vi "多通道CAN FD回读.vi"(8 "错误输入（无错误）":errorcluster, 10 "Delay Time (s)":dbl=0.2 format="%#_13g", 11 "CAN通道in":u16[](array[numeric])=[81, 82, 83]) -> (0 "错误输出":errorcluster, 3 "报文数组":string[](array[string]))   [LabVIEW 2021]
panel:
  out "function return":u32
  in  "MessageBuffer in":T1 {"DATA"."[0]" format="%x"; "DATA"."[1]" format="%x"; "DATA"."[2]" format="%x"; "DATA"."[3]" format="%x"; "DATA"."[4]" format="%x"; "DATA"."[5]" format="%x"; "DATA"."[6]" format="%x"; "DATA"."[7]" format="%x"; "DATA"."[8]" format="%x"; "DATA"."[9]" format="%x"; "DATA"."[10]" format="%x"; "DATA"."[11]" format="%x"; "DATA"."[12]" format="%x"; "DATA"."[13]" format="%x"; "DATA"."[14]" format="%x"; "DATA"."[15]" format="%x"; "DATA"."[16]" format="%x"; "DATA"."[17]" format="%x"; "DATA"."[18]" format="%x"; "DATA"."[19]" format="%x"; "DATA"."[20]" format="%x"; "DATA"."[21]" format="%x"; "DATA"."[22]" format="%x"; "DATA"."[23]" format="%x"; "DATA"."[24]" format="%x"; "DATA"."[25]" format="%x"; "DATA"."[26]" format="%x"; "DATA"."[27]" format="%x"; "DATA"."[28]" format="%x"; "DATA"."[29]" format="%x"; "DATA"."[30]" format="%x"; "DATA"."[31]" format="%x"; "DATA"."[32]" format="%x"; "DATA"."[33]" format="%x"; "DATA"."[34]" format="%x"; "DATA"."[35]" format="%x"; "DATA"."[36]" format="%x"; "DATA"."[37]" format="%x"; "DATA"."[38]" format="%x"; "DATA"."[39]" format="%x"; "DATA"."[40]" format="%x"; "DATA"."[41]" format="%x"; "DATA"."[42]" format="%x"; "DATA"."[43]" format="%x"; "DATA"."[44]" format="%x"; "DATA"."[45]" format="%x"; "DATA"."[46]" format="%x"; "DATA"."[47]" format="%x"; "DATA"."[48]" format="%x"; "DATA"."[49]" format="%x"; "DATA"."[50]" format="%x"; "DATA"."[51]" format="%x"; "DATA"."[52]" format="%x"; "DATA"."[53]" format="%x"; "DATA"."[54]" format="%x"; "DATA"."[55]" format="%x"; "DATA"."[56]" format="%x"; "DATA"."[57]" format="%x"; "DATA"."[58]" format="%x"; "DATA"."[59]" format="%x"; "DATA"."[60]" format="%x"; "DATA"."[61]" format="%x"; "DATA"."[62]" format="%x"; "DATA"."[63]" format="%x"; "ID" format="%.0x"; "MSGTYPE" format="%.0x"; "DLC" format="%.0x"}
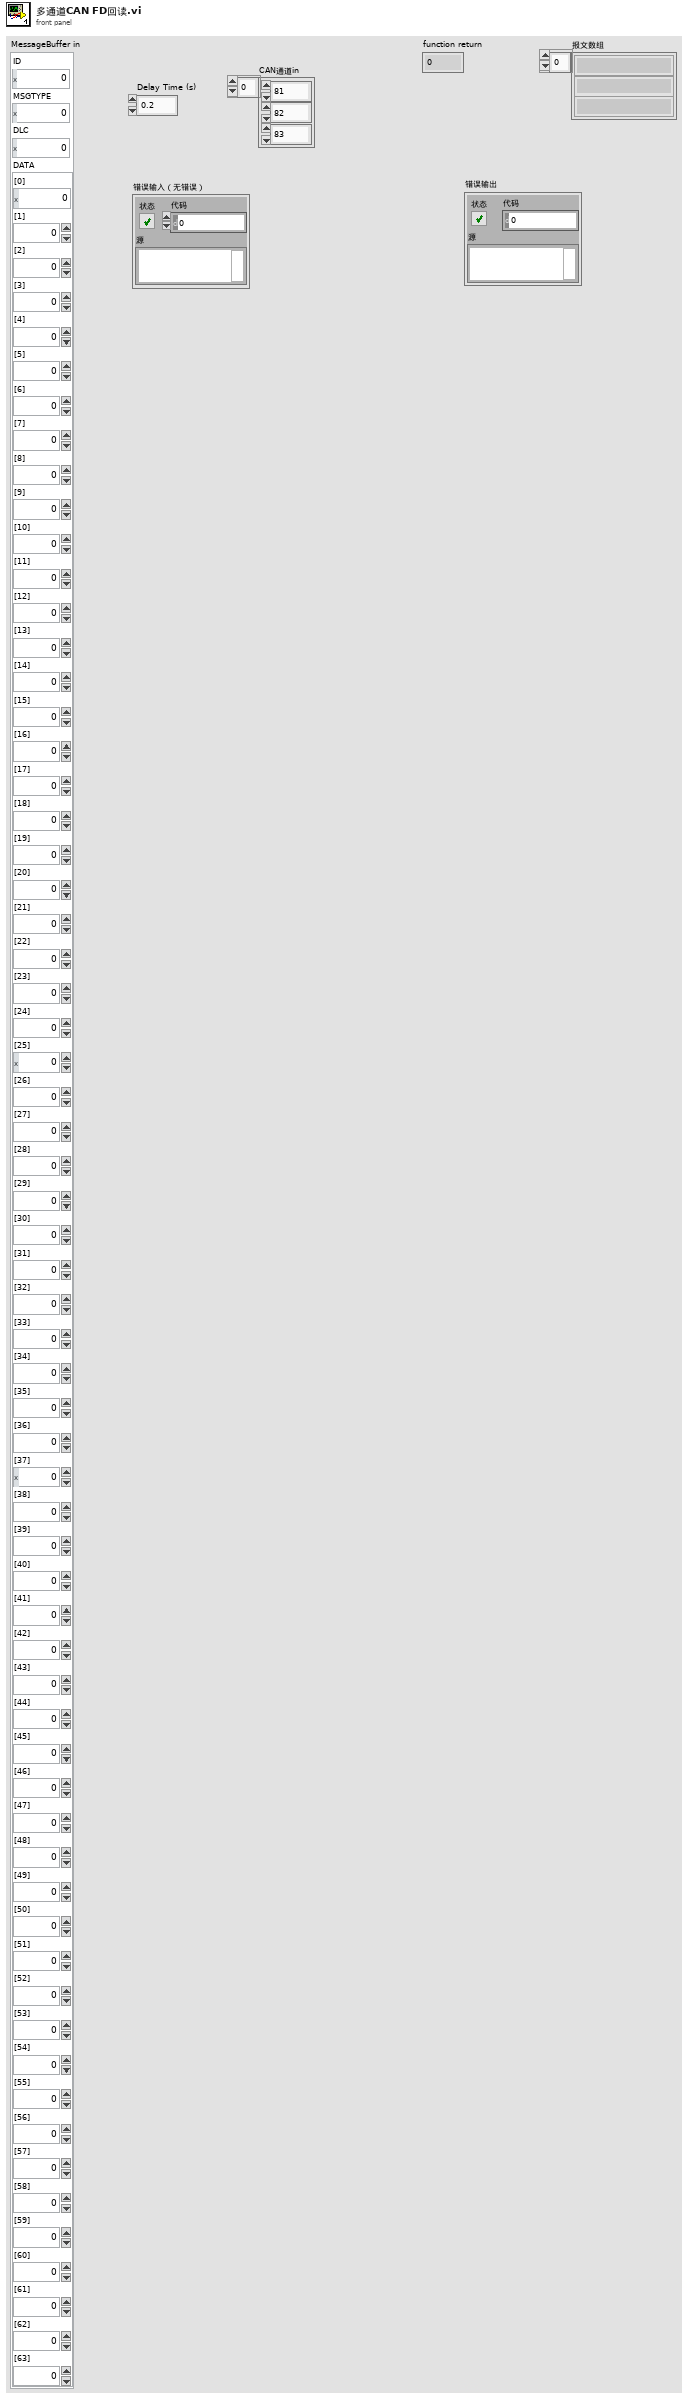
[diagram p1: front panel]
types:
  T1 = cluster{"ID":u32, "MSGTYPE":u8, "DLC":u8, "DATA":cluster{"[0]":u8, "[1]":u8, "[2]":u8, "[3]":u8, "[4]":u8, "[5]":u8, "[6]":u8, "[7]":u8, "[8]":u8, "[9]":u8, "[10]":u8, "[11]":u8, "[12]":u8, "[13]":u8, "[14]":u8, "[15]":u8, "[16]":u8, "[17]":u8, "[18]":u8, "[19]":u8, "[20]":u8, "[21]":u8, "[22]":u8, "[23]":u8, "[24]":u8, "[25]":u8, "[26]":u8, "[27]":u8, "[28]":u8, "[29]":u8, "[30]":u8, "[31]":u8, "[32]":u8, "[33]":u8, "[34]":u8, "[35]":u8, "[36]":u8, "[37]":u8, "[38]":u8, "[39]":u8, "[40]":u8, "[41]":u8, "[42]":u8, "[43]":u8, "[44]":u8, "[45]":u8, "[46]":u8, "[47]":u8, "[48]":u8, "[49]":u8, "[50]":u8, "[51]":u8, "[52]":u8, "[53]":u8, "[54]":u8, "[55]":u8, "[56]":u8, "[57]":u8, "[58]":u8, "[59]":u8, "[60]":u8, "[61]":u8, "[62]":u8, "[63]":u8}}
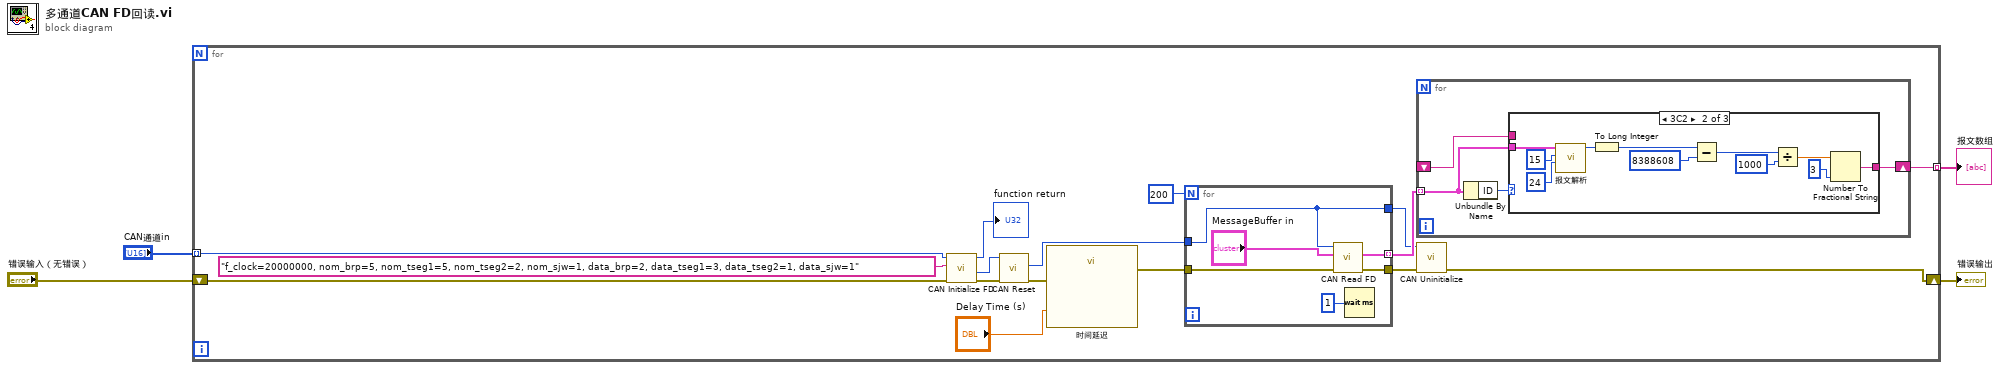
[diagram p0: block diagram]
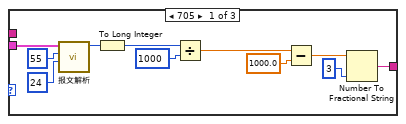
[diagram p2: hidden frame]
diagram:
  n1 = for {
    tunnel: "CAN通道in" -> [w12] mode=indexing
    shift-right: [w10] -> w3
    shift-left: "错误输入（无错误）" -> [w8]
    tunnel: [w9] -> w1 mode=indexing
    n2 = call "CAN Initialize FD.vi"("错误输入（无错误）"=w8, "BitrateFD"="f_clock=20000000, nom_brp=5, nom_tseg1=5, nom_tseg2=2, nom_sjw=1, data_brp=2, data_tseg1=3, data_tseg2=1, data_sjw=1", "Channel"=w12) -> ("错误输出"=w7:errorcluster, "Channel out"=w11:u16, "function return"=→"function return":u32)  [unwired: 5 in, 1 out]
    n3 = call "CAN Reset.vi"("错误输入（无错误）"=w7, "Channel in"=w11) -> ("错误输出"=w15:errorcluster, "Channel out"=w17:u16)  [unwired: 7 in, 1 out]
    n4 = call "时间延迟"("error in (no error)"=w15, "Delay Time (s)"="Delay Time (s)") -> ("error out"=w14:errorcluster)  [unwired: 9 in]
    n5 = for {
      N: 200 -> [_]
      tunnel: w17 -> [w51]
      tunnel: [w52] -> w19 mode=indexing
      tunnel: [w51] -> w18
      tunnel: w14 -> [w50]
      tunnel: [w49] -> w16
      n6 = call "CAN Read FD.vi"("error in (no error)"=w50, "MessageBuffer in"="MessageBuffer in", "Channel"=w51) -> ("error out"=w49:errorcluster, "MessageBuffer out"=w52:T1)  [unwired: 5 in, 2 out]
      n7 = Wait (ms)(milliseconds to wait=u32 1 ("等待时间（毫秒）")) -> ()  [unwired: 1 out]
    }
    n8 = for {
      tunnel: w19 -> [w23] mode=indexing
      shift-right: [w22] -> w9
      shift-left: _ -> [w21]
      n9 = Unbundle By Name(w23) -> ("ID"=w24:u32)
      n10 = case shown="3C2" w24 {
        tunnel: w23 -> [w35 w44 _]
        tunnel: [w32 w36 w47] -> w22
        tunnel: w21 -> [_ _ w47]
        frame 705 {
          n11 = call "报文解析.vi"("长度"=24, "起始位"=55, "MessageBuffer in"=w35) -> ("数字"=w31:u32)  [unwired: 8 in]
          n12 = To Long Integer(number=w31) -> (32bit integer=w30:i32)
          n13 = Divide(x=w30, y=1000) -> (x/y=w28:dbl)
          n14 = Subtract(x=w28, y=1000.0) -> (x-y=w26:dbl)
          n15 = Number To Fractional String(number=w26, precision (6)=i16 3 ("宽度(-)")) -> (F-format string=w32:string)  [unwired: 2 in]
        }
        frame 962 {
          n16 = call "报文解析.vi"("长度"=24, "起始位"=15, "MessageBuffer in"=w44) -> ("数字"=w42:u32)  [unwired: 8 in]
          n17 = To Long Integer(number=w42) -> (32bit integer=w41:i32)
          n18 = Subtract(x=w41, y=8388608) -> (x-y=w40:i32)
          n19 = Divide(x=w40, y=1000) -> (x/y=w38:dbl)
          n20 = Number To Fractional String(number=w38, precision (6)=i16 3 ("精度(6)")) -> (F-format string=w36:string)  [unwired: 2 in]
        }
        frame 770, Default {
        }
      }
    }
    n21 = call "CAN Uninitialize.vi"("错误输入（无错误）"=w16, "Channel"=w18) -> ("错误输出"=w10:errorcluster)  [unwired: 7 in, 2 out]
  }
  "错误输出" <- w3
  "报文数组" <- w1
